vi "ConfigClkRef.vi"(8 "error in (no error)":errorcluster, 11 "PXI_MultiTrig in":refnum<class "PXI_MultiTrig.lvclass">) -> (0 "error out":errorcluster, 3 "PXI_MultiTrig out":refnum<class "PXI_MultiTrig.lvclass">)   [LabVIEW 2018, in "SyncPlugins.lvlib" / "PXI_MultiTrig.lvclass"]
uses:
  PXI_MultiTrig.lvclass
  PXI_MultiTrig.lvclass/PXI_MultiTrig.ctl
  Accessors/Read TimeRefType.vi
  Accessors/Read RefClkHandle.vi
  Accessors/Write RefClkSession.vi
  <instrlib>/niSync/niSync.llb/niSync Initialize (IVI).vi
  <instrlib>/niSync/niSync.llb/niSync Set Time Reference (1588 Ordinary Clock).vi
  <instrlib>/niSync/niSync.llb/niSync Set Time Reference (Free Running).vi
  <instrlib>/niSync/niSync.llb/niSync Set Time Reference (GPS).vi
  <instrlib>/niSync/niSync.llb/niSync Set Time Reference (IRIG).vi
  <instrlib>/niSync/niSync.llb/niSync Set Time Reference (PPS).vi
  <vilib>/Utility/error.llb/Error Cluster From Error Code.vi
  <vilib>/ErrorRing/Error Ring.xnode
panel:
  out "GPS:Status":i32(ring) items=["Uninitialized", "Antenna Error", "No Useable Satellites", "One Useable Satellite", "Two Useable Satellites", "Three Useable Satellites", "No GPS Time", "PDOP Too High", "Unusable Satellite", "Fix Rejected", "Self Survey Complete", "Self Survey Not Complete"]
  out "1588:Clock State":i32(ring) items=["Initializing", "Faulty", "Disabled", "Listening", "PreMaster", "Master", "Passive", "Uncalibrated", "Slave", "Stopped"]
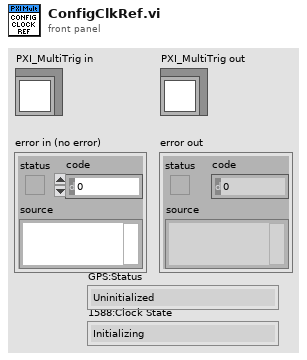
[diagram p1: front panel]
types:
  T1 = typedef "SyncPlugins.lvlib/PXI_MultiTrig.lvclass/TimeRefType.ctl" = enum16{"1588", "Free Running", "GPS", "IRIG", "PPS"}
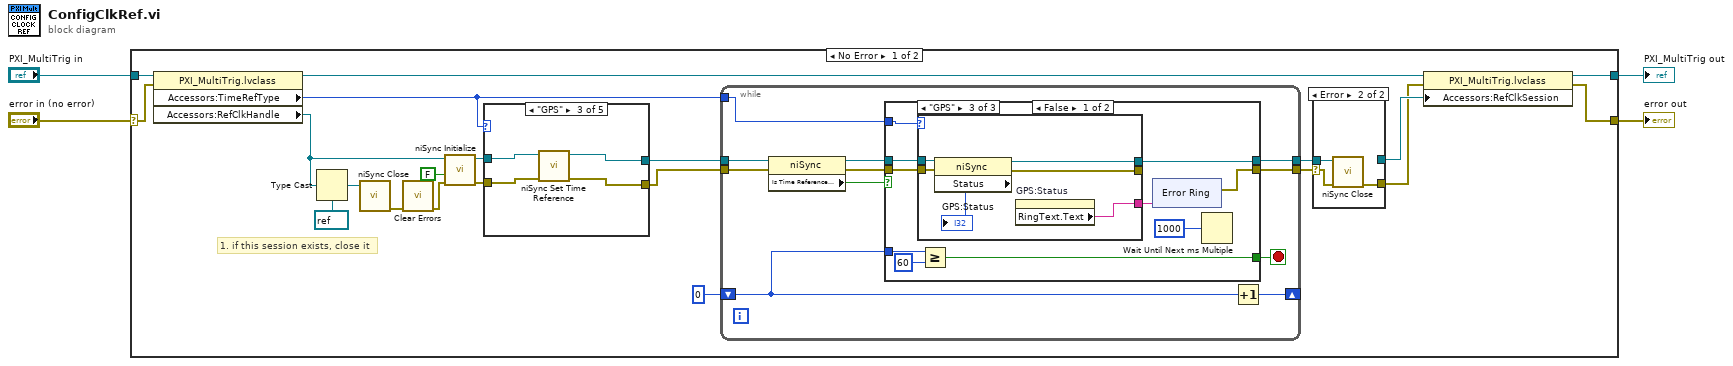
[diagram p0: block diagram]
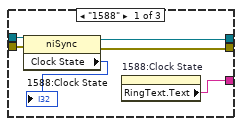
[diagram p3: hidden frame]
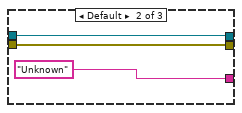
[diagram p4: hidden frame]
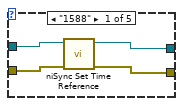
[diagram p6: hidden frame]
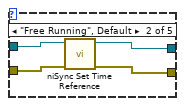
[diagram p7: hidden frame]
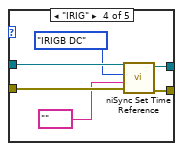
[diagram p8: hidden frame]
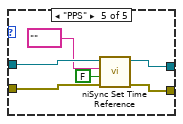
[diagram p9: hidden frame]
diagram:
  n1 = case shown="No Error" "error in (no error)" {
    selector: "error in (no error)" -> [w23 w102]
    tunnel: [w22 w102] -> w3
    tunnel: [w24 w101] -> w1
    tunnel: "PXI_MultiTrig in" -> [w25 w101]
    frame No Error {
      # "1. if this session exists, close it"
      n2 = property class="PXI_MultiTrig.lvclass"(reference=w25, error in=w23) -> (reference out=w18:refnum<class "PXI_MultiTrig.lvclass">, "Accessors:TimeRefType"=w15:T1, "Accessors:RefClkHandle"=w8:refnum<k15>)  [unwired: 1 out]
      n3 = Type Cast(type=refnum<k15> refnum ("instrument handle"), x=w8) -> (*(type *) &x=w9:refnum<k15>)
      n4 = call <instrlib>:"niSync Close.vi"("instrument handle"=w9) -> ("error out"=w7:errorcluster)  [unwired: 10 in]
      n5 = call <vilib>:"Clear Errors.vi"("error in (no error)"=w7) -> ("error out"=w6:errorcluster)  [unwired: 5 in, 1 out]
      n6 = call-poly <instrlib>:"niSync Initialize.vi"("error in (no error)"=w6, "reset device (F)"=FALSE, "resource name"=w8) -> ("error out"=w19:errorcluster, "instrument handle out"=w21:refnum<k15>)  [unwired: 7 in]
      n7 = case shown="\"GPS\"" w15 {
        tunnel: w21 -> [w80 w84 w88 w94 w100]
        tunnel: w19 -> [w79 w83 w87 w93 w99]
        tunnel: [w78 w82 w86 w92 w98] -> w20
        tunnel: [w77 w81 w85 w91 w97] -> w17
        frame "1588" {
          n8 = call-poly <instrlib>:"niSync Set Time Reference.vi"("error in (no error)"=w79, "instrument handle"=w80) -> ("error out"=w77:errorcluster, "instrument handle out"=w78:refnum<k15>)  [unwired: 8 in]
        }
        frame "Free Running", Default {
          n9 = call-poly <instrlib>:"niSync Set Time Reference.vi"("error in (no error)"=w83, "instrument handle"=w84) -> ("error out"=w81:errorcluster, "instrument handle out"=w82:refnum<k15>)  [unwired: 8 in]
        }
        frame "GPS" {
          n10 = call-poly <instrlib>:"niSync Set Time Reference.vi"("error in (no error)"=w87, "instrument handle"=w88) -> ("error out"=w85:errorcluster, "instrument handle out"=w86:refnum<k15>)  [unwired: 8 in]
        }
        frame "IRIG" {
          n11 = call-poly <instrlib>:"niSync Set Time Reference.vi"("error in (no error)"=w93, "terminal"=tag "", "IRIG type"=enum16{"IRIGB DC", "IRIGB AM"}."IRIGB DC", "instrument handle"=w94) -> ("error out"=w91:errorcluster, "instrument handle out"=w92:refnum<k15>)  [unwired: 6 in]
        }
        frame "PPS" {
          n12 = call-poly <instrlib>:"niSync Set Time Reference.vi"("error in (no error)"=w99, "use manual time"=FALSE, "terminal"=tag "", "instrument handle"=w100) -> ("error out"=w97:errorcluster, "instrument handle out"=w98:refnum<k15>)  [unwired: 6 in]
        }
      }
      n13 = while {
        tunnel: w20 -> [w41]
        tunnel: w17 -> [w40]
        shift-right: [w38] -> _
        shift-left: 0 -> [w32]
        tunnel: [w34] -> w12
        tunnel: [w33] -> w11
        tunnel: w15 -> [w31]
        stop <- w37 stop-if-true
        n14 = property class="niSync"(reference=w41, error in=w40) -> (reference out=w36:refnum<k15>, error out=w35:errorcluster, "Is Time Reference Present"=w39:bool)
        n15 = case shown="False" w39 {
          selector: w39 -> [_ w76]
          tunnel: [w48 w76] -> w37
          tunnel: w36 -> [w47 w75]
          tunnel: w35 -> [w46 w74]
          tunnel: [w45 w75] -> w34
          tunnel: [w42 w74] -> w33
          tunnel: w32 -> [w51 _]
          tunnel: w31 -> [w44 _]
          frame False {
            n16 = case shown="\"GPS\"" w44 {
              tunnel: w47 -> [w64 w67 w73]
              tunnel: w46 -> [w63 w66 w72]
              tunnel: [w62 w67 w71] -> w45
              tunnel: [w61 w66 w70] -> _
              tunnel: [w59 "Unknown" w68] -> w43
              frame "1588" {
                n17 = property class="niSync"(reference=w64, error in=w63) -> (reference out=w62:refnum<k15>, error out=w61:errorcluster, "Clock State"=→"1588:Clock State":i32)
                n18 = property on="1588:Clock State" class="Ring (strict)"() -> ("RingText.Text"=w59:string)  [unwired: 2 in, 2 out]
              }
              frame Default {
              }
              frame "GPS" {
                n19 = property class="niSync"(reference=w73, error in=w72) -> (reference out=w71:refnum<k15>, error out=w70:errorcluster, "Status"=→"GPS:Status":i32)
                n20 = property on="GPS:Status" class="Ring (strict)"() -> ("RingText.Text"=w68:string)  [unwired: 2 in, 2 out]
              }
            }
            n21 = Greater Or Equal?(x=w51, y=60) -> (x >= y?=w48:bool)
            n22 = xnode "Error Ring"("parameter 0"=w43) -> ("error out"=w42:errorcluster)
            n23 = Wait Until Next ms Multiple(millisecond multiple=u32 1000) -> ()  [unwired: 1 out]
          }
          frame True {
          }
        }
        n24 = Increment(x=w32) -> (x+1=w38:i32)
      }
      n25 = case shown="Error" w11 {
        selector: w11 -> [w26 w29]
        tunnel: w12 -> [w27 w30]
        tunnel: [w27 _] -> w14
        tunnel: [w26 w28] -> w13
        frame No Error {
        }
        frame Error {
          n26 = call <instrlib>:"niSync Close.vi"("error in (no error)"=w29, "instrument handle"=w30) -> ("error out"=w28:errorcluster)  [unwired: 9 in]
        }
      }
      n27 = property class="PXI_MultiTrig.lvclass"(reference=w18, error in=w13, "Accessors:RefClkSession"=w14) -> (reference out=w24:refnum<class "PXI_MultiTrig.lvclass">, error out=w22:errorcluster)
    }
    frame Error {
    }
  }
  "error out" <- w3
  "PXI_MultiTrig out" <- w1
